vi "Ex. 1 Front panel objects.vi"() -> ()   [LabVIEW 2024]
panel:
  out "String 2":string
  in  "String":string
  out "Boolean":bool
  in  "Stop":bool
  out "Numeric 2":dbl
  in  "Numeric":dbl
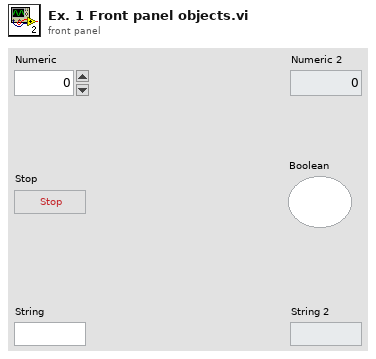
[diagram p1: front panel]
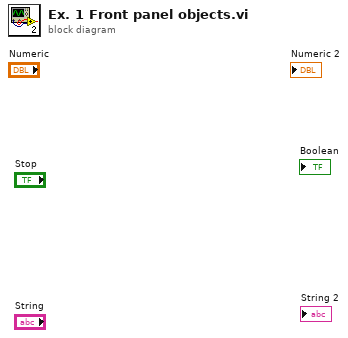
[diagram p0: block diagram]
diagram:
